vi "Ch_data_pattern_16_save (SubVI).vi"(7 "error in":errorcluster, 10 "R1-8 Cluster":T1, 12 "T1-8 Cluster":T2, 14 "R9-16":T1, 15 "Activate!":bool, 16 "T9-16":T2, 17 "file":refnum<file>) -> (27 "error out":errorcluster)   [LabVIEW 8.6]
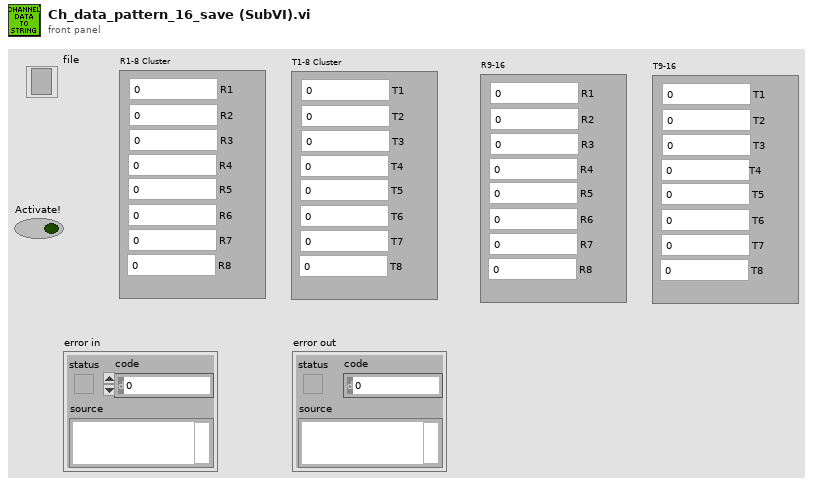
[diagram p1: front panel]
types:
  T1 = cluster{"R1":dbl, "R2":dbl, "R3":dbl, "R4":dbl, "R5":dbl, "R6":dbl, "R7":dbl, "R8":dbl}
  T2 = cluster{"T1":dbl, "T2":dbl, "T3":dbl, "T4":dbl, "T5":dbl, "T6":dbl, "T7":dbl, "T8":dbl}
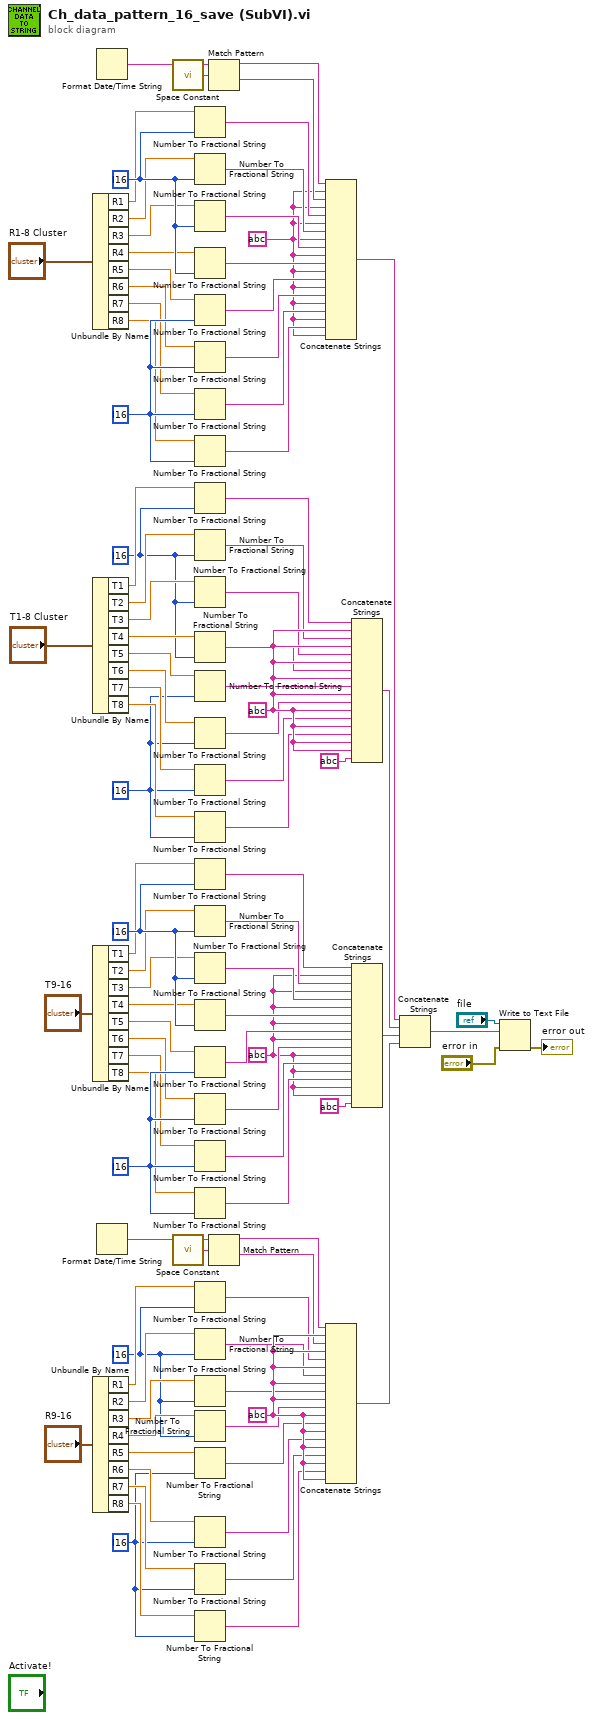
[diagram p0: block diagram]
diagram:
  w39 = i16 ? ("precision (6)")
  w43 = i16 ? ("precision (6)")
  w26 = string ?
  w12 = i16 ? ("precision (6)")
  w3 = i16 ? ("precision (6)")
  w25 = string ?
  w58 = i16 ? ("precision (6)")
  w54 = i16 ? ("precision (6)")
  w71 = string ?
  w87 = i16 ? ("precision (6)")
  w97 = i16 ? ("precision (6)")
  w74 = string ?
  n1 = Unbundle By Name("R1-8 Cluster") -> ("R1"=w82:dbl, "R2"=w81:dbl, "R3"=w80:dbl, "R4"=w79:dbl, "R5"=w78:dbl, "R6"=w77:dbl, "R7"=w76:dbl, "R8"=w75:dbl)
  n2 = Unbundle By Name("T1-8 Cluster") -> ("T1"=w63:dbl, "T2"=w64:dbl, "T3"=w65:dbl, "T4"=w66:dbl, "T5"=w67:dbl, "T6"=w68:dbl, "T7"=w69:dbl, "T8"=w70:dbl)
  n3 = Unbundle By Name("T9-16") -> ("T1"=w34:dbl, "T2"=w33:dbl, "T3"=w32:dbl, "T4"=w31:dbl, "T5"=w30:dbl, "T6"=w29:dbl, "T7"=w28:dbl, "T8"=w27:dbl)
  n4 = Unbundle By Name("R9-16") -> ("R1"=w17:dbl, "R2"=w18:dbl, "R3"=w19:dbl, "R4"=w20:dbl, "R5"=w21:dbl, "R6"=w22:dbl, "R7"=w23:dbl, "R8"=w24:dbl)
  n5 = Format Date/Time String() -> (date/time string=w89:string)  [unwired: 3 out]
  n6 = Format Date/Time String() -> (date/time string=w11:string)  [unwired: 3 out]
  n7 = call <vilib>:"Space Constant.vi"() -> ("String"=w90:string)
  n8 = call <vilib>:"Space Constant.vi"() -> ("String"=w10:string)
  n9 = Number To Fractional String(number=w82, precision (6)=w97) -> (F-format string=w93:string)  [unwired: 2 out]
  n10 = Number To Fractional String(number=w81, precision (6)=w97) -> (F-format string=w94:string)  [unwired: 2 out]
  n11 = Number To Fractional String(number=w80, precision (6)=w97) -> (F-format string=w95:string)  [unwired: 2 out]
  n12 = Number To Fractional String(number=w79, precision (6)=w97) -> (F-format string=w96:string)  [unwired: 2 out]
  n13 = Number To Fractional String(number=w78, precision (6)=w87) -> (F-format string=w86:string)  [unwired: 2 out]
  n14 = Number To Fractional String(number=w77, precision (6)=w87) -> (F-format string=w85:string)  [unwired: 2 out]
  n15 = Number To Fractional String(number=w76, precision (6)=w87) -> (F-format string=w84:string)  [unwired: 2 out]
  n16 = Number To Fractional String(number=w75, precision (6)=w87) -> (F-format string=w83:string)  [unwired: 2 out]
  n17 = Number To Fractional String(number=w63, precision (6)=w54) -> (F-format string=w57:string)  [unwired: 2 out]
  n18 = Number To Fractional String(number=w64, precision (6)=w54) -> (F-format string=w50:string)  [unwired: 2 out]
  n19 = Number To Fractional String(number=w65, precision (6)=w54) -> (F-format string=w56:string)  [unwired: 2 out]
  n20 = Number To Fractional String(number=w66, precision (6)=w54) -> (F-format string=w55:string)  [unwired: 2 out]
  n21 = Number To Fractional String(number=w67, precision (6)=w58) -> (F-format string=w59:string)  [unwired: 2 out]
  n22 = Number To Fractional String(number=w68, precision (6)=w58) -> (F-format string=w60:string)  [unwired: 2 out]
  n23 = Number To Fractional String(number=w69, precision (6)=w58) -> (F-format string=w61:string)  [unwired: 2 out]
  n24 = Number To Fractional String(number=w70, precision (6)=w58) -> (F-format string=w62:string)  [unwired: 2 out]
  n25 = Number To Fractional String(number=w34, precision (6)=w43) -> (F-format string=w40:string)  [unwired: 2 out]
  n26 = Number To Fractional String(number=w33, precision (6)=w43) -> (F-format string=w45:string)  [unwired: 2 out]
  n27 = Number To Fractional String(number=w32, precision (6)=w43) -> (F-format string=w41:string)  [unwired: 2 out]
  n28 = Number To Fractional String(number=w31, precision (6)=w43) -> (F-format string=w42:string)  [unwired: 2 out]
  n29 = Number To Fractional String(number=w30, precision (6)=w39) -> (F-format string=w38:string)  [unwired: 2 out]
  n30 = Number To Fractional String(number=w29, precision (6)=w39) -> (F-format string=w37:string)  [unwired: 2 out]
  n31 = Number To Fractional String(number=w28, precision (6)=w39) -> (F-format string=w36:string)  [unwired: 2 out]
  n32 = Number To Fractional String(number=w27, precision (6)=w39) -> (F-format string=w35:string)  [unwired: 2 out]
  n33 = Number To Fractional String(number=w17, precision (6)=w3) -> (F-format string=w7:string)  [unwired: 2 out]
  n34 = Number To Fractional String(number=w18, precision (6)=w3) -> (F-format string=w6:string)  [unwired: 2 out]
  n35 = Number To Fractional String(number=w19, precision (6)=w3) -> (F-format string=w5:string)  [unwired: 2 out]
  n36 = Number To Fractional String(number=w20, precision (6)=w3) -> (F-format string=w4:string)  [unwired: 2 out]
  n37 = Number To Fractional String(number=w21, precision (6)=w12) -> (F-format string=w13:string)  [unwired: 2 out]
  n38 = Number To Fractional String(number=w22, precision (6)=w12) -> (F-format string=w14:string)  [unwired: 2 out]
  n39 = Number To Fractional String(number=w23, precision (6)=w12) -> (F-format string=w15:string)  [unwired: 2 out]
  n40 = Number To Fractional String(number=w24, precision (6)=w12) -> (F-format string=w16:string)  [unwired: 2 out]
  n41 = Match Pattern(string=w89, regular expression=w90) -> (before substring=w91:string, after substring=w92:string)  [unwired: 3 out]
  n42 = Match Pattern(string=w11, regular expression=w10) -> (before substring=w9:string, after substring=w8:string)  [unwired: 3 out]
  n43 = Concatenate Strings(w91, w74, w92, w74, w93, w74, w94, w74, w95, w74, w96, w74, w86, w74, w85, w74, w84, w74, w83, w74) -> (w73:string)
  n44 = Concatenate Strings(w9, w25, w8, w25, w7, w25, w6, w25, w5, w25, w4, w25, w13, w25, w14, w25, w15, w25, w16, w25) -> (w1:string)
  n45 = Concatenate Strings(w57, w71, w50, w71, w56, w71, w55, w71, w59, w71, w60, w71, w61, w71, w62, w71, w71, string ?) -> (w52:string)
  n46 = Concatenate Strings(w40, w26, w45, w26, w41, w26, w42, w26, w38, w26, w37, w26, w36, w26, w35, w26, w26, string ?) -> (w2:string)
  n47 = Concatenate Strings(w73, w52, w2, w1) -> (w72:string)
  n48 = Write to Text File(file (use dialog)="file", text=w72, error in="error in") -> (error out=→"error out":errorcluster)  [unwired: 3 out]
